vi "CommandPickup.vi"(10 "Gripper Value":dbl, 11 "Elevator Value":dbl) -> (3 "appended array":cluster{"States":T1, "Numeric":dbl}[](array[cluster]))   [LabVIEW 2014, in "Elevator System.lvlib"]
uses:
  Elevator System.lvlib
  Typedef/ControllerStates.ctl
  Typedef/TeirNumber.ctl
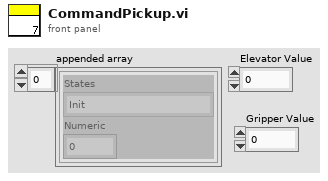
[diagram p1: front panel]
types:
  T1 = typedef "Elevator System.lvlib/ControllerStates.ctl" = enum16{"Init", "Set Elevator SP", "Set Gripper SP", "Wait For Elevator", "Wait For Gripper", ""}
  T2 = typedef "Elevator System.lvlib/TeirNumber.ctl" = enum16{"T1", "T2", "T3", "T4", "T5", "T6"}
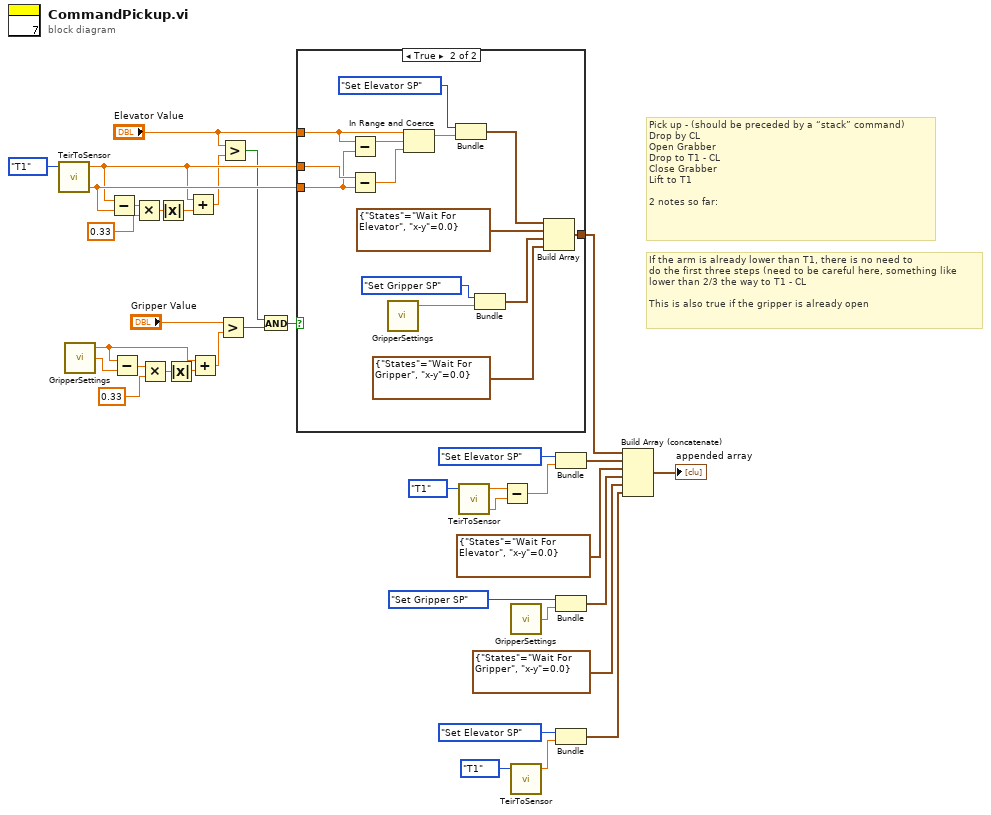
[diagram p0: block diagram]
diagram:
  # "If the arm is already lower than T1, there is no need to \ndo the first three steps (need to be careful here, something like \nlower than 2/3 the way to T1 - CL \n\nThis is also true if the gripper is already open"
  # "Pick up - (should be preceded by a “stack” command)\nDrop by CL\nOpen Grabber\nDrop to T1 - CL\nClose Grabber\nLift to T1\n\n2 notes so far:"
  n1 = call "TeirToSensor.vi"("Enum"=TeirNumber."T1") -> ("CL"=w18:dbl, "Numeric"=w14:dbl)  [unwired: 2 in, 1 out]
  n2 = call "GripperSettings.vi"() -> ("Open"=w10:dbl, "Close"=w5:dbl)  [unwired: 2 in, 1 out]
  n3 = Subtract(x=w14, y=w18) -> (x-y=w17:dbl)
  n4 = Subtract(x=w10, y=w5) -> (x-y=w6:dbl)
  n5 = Multiply(x=w17, y=0.33) -> (x*y=w15:dbl)
  n6 = Multiply(x=w6, y=0.33) -> (x*y=w8:dbl)
  n7 = Absolute Value(x=w15) -> (abs(x)=w12:dbl)
  n8 = Absolute Value(x=w8) -> (abs(x)=w9:dbl)
  n9 = Add(x=w14, y=w12) -> (x+y=w13:dbl)
  n10 = Add(x=w10, y=w9) -> (x+y=w11:dbl)
  n11 = Greater?(x="Gripper Value", y=w11) -> (0:w1:bool)
  n12 = Greater?(x="Elevator Value", y=w13) -> (0:w2:bool)
  n13 = And(x=w2, y=w1) -> (x .and. y?=w3:bool)
  n14 = case shown="True" w3 {
    tunnel: w14 -> [_ w49]
    tunnel: w18 -> [_ w48]
    tunnel: "Elevator Value" -> [_ w46]
    tunnel: [_ w40] -> w19
    frame False {
    }
    frame True {
      n15 = Subtract(x=w46, y=w48) -> (x-y=w50:dbl)
      n16 = Subtract(x=w49, y=w48) -> (x-y=w47:dbl)
      n17 = call "GripperSettings.vi"() -> ("Open"=w38:dbl)  [unwired: 2 in, 2 out]
      n18 = In Range and Coerce(upper limit=w46, x=w50, lower limit=w47) -> (coerced(x)=w45:dbl)  [unwired: 1 out]
      n19 = Bundle("States"=ControllerStates."Set Elevator SP", "Elevator Value"=w45) -> (w44:cluster{"States":T1, "Elevator Value":dbl})  [unwired: 1 in]
      n20 = Bundle("States"=ControllerStates."Set Gripper SP", "Open"=w38) -> (w42:cluster{"States":T1, "Open":dbl})  [unwired: 1 in]
      n21 = Build Array(w44, cluster{"States":T1, "x-y":dbl} {"States"=enum."Wait For Elevator", "x-y"=0.0}, w42, cluster{"States":T1, "x-y":dbl} {"States"=enum."Wait For Gripper", "x-y"=0.0}) -> (w40:cluster{"States":T1, "x-y":dbl}[])
    }
  }
  n22 = call "TeirToSensor.vi"("Enum"=TeirNumber."T1") -> ("CL"=w32:dbl, "Numeric"=w31:dbl)  [unwired: 2 in, 1 out]
  n23 = Subtract(x=w31, y=w32) -> (x-y=w29:dbl)
  n24 = call "GripperSettings.vi"() -> ("Close"=w24:dbl)  [unwired: 2 in, 2 out]
  n25 = call "TeirToSensor.vi"("Enum"=TeirNumber."T1") -> ("Numeric"=w34:dbl)  [unwired: 2 in, 2 out]
  n26 = Bundle("States"=ControllerStates."Set Elevator SP", w29) -> (w27:cluster{"States":T1, dbl})  [unwired: 1 in]
  n27 = Bundle("States"=ControllerStates."Set Gripper SP", "Close"=w24) -> (w25:cluster{"States":T1, "Close":dbl})  [unwired: 1 in]
  n28 = Bundle("States"=ControllerStates."Set Elevator SP", "Numeric"=w34) -> (w36:cluster{"States":T1, "Numeric":dbl})  [unwired: 1 in]
  n29 = Build Array (concatenate)(w19, w27, cluster{"States":T1, "x-y":dbl} {"States"=enum."Wait For Elevator", "x-y"=0.0}, w25, cluster{"States":T1, "x-y":dbl} {"States"=enum."Wait For Gripper", "x-y"=0.0}, w36) -> (→"appended array":cluster{"States":T1, "Numeric":dbl}[])
